vi "Array Average Polymorphic.vi"   [LabVIEW 2014]
doc: "This polymorphic VI takes in an array and calculate the average, min, and max"
uses:
  Labview Reliability Implementation/Linear Regression/Linear Regression.lvlib
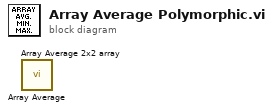
[diagram p0: block diagram]
diagram:
  n1 = call "Array Average.vi"() -> ()  [unwired: 3 in, 3 out]
  n2 = call "Array Average 2x2 array.vi"() -> ()  [unwired: 3 in, 3 out]
